vi "To Wiki Name.vi"(3 "Name":string) -> (1 "Wiki Name":string)   [LabVIEW 2014]
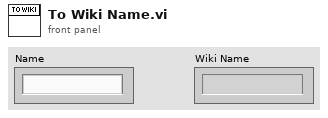
[diagram p1: front panel]
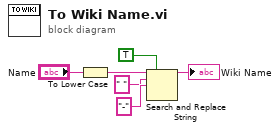
[diagram p0: block diagram]
diagram:
  n1 = To Lower Case(string="Name") -> (all lower case string=w4:string)
  n2 = Search and Replace String(replace all?=TRUE ("replace all? (F)"), input string=w4, search string=" ", replace string="-" ("replace string (\"\")")) -> (result string=→"Wiki Name":string)  [unwired: 4 in, 3 out]
